vi "RT Positions.vi"(1 "Coordinates":dbl[][](array[numeric]) format="%.6f", 2 "L/R":bool) -> (0 "Cluster":T2)   [LabVIEW 2010]
uses:
  <vilib>/Analysis/Matrix/Datatypes/RealMatrix.ctl
  <vilib>/Analysis/baseanly.llb/Real A x B.vi
  <vilib>/Analysis/NI_AALBase.lvlib
  <vilib>/Analysis/Matrix/NI_Matrix.lvlib
panel:
  out "Humerus rel Trunk":T1
  out "[R]T Trunk":dbl[][](array[numeric])
  out "[R] Trunk":dbl[][](array[numeric])
  out "[R]T Forearm":dbl[][](array[numeric])
  out "[R] Forearm":dbl[][](array[numeric])
  out "[R]T Humerus":dbl[][](array[numeric])
  out "[R] Humerus":dbl[][](array[numeric])
  out "EJC Coord":dbl[](array[numeric])
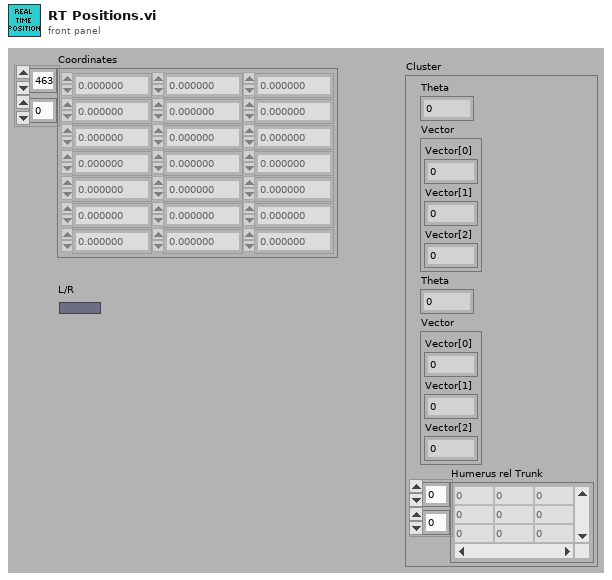
[diagram p1: front panel]
types:
  T1 = typedef "NI_Matrix.lvlib/RealMatrix.ctl" = dbl[][]
  T2 = cluster{"Theta":dbl, "Vector":cluster{"Vector[0]":ext, "Vector[1]":ext, "Vector[2]":ext}, "Theta":dbl, "Vector":cluster{"Vector[0]":ext, "Vector[1]":ext, "Vector[2]":ext}, "Humerus rel Trunk":T1}
  T3 = cluster{"Vector[0]":ext, "Vector[1]":ext, "Vector[2]":ext}
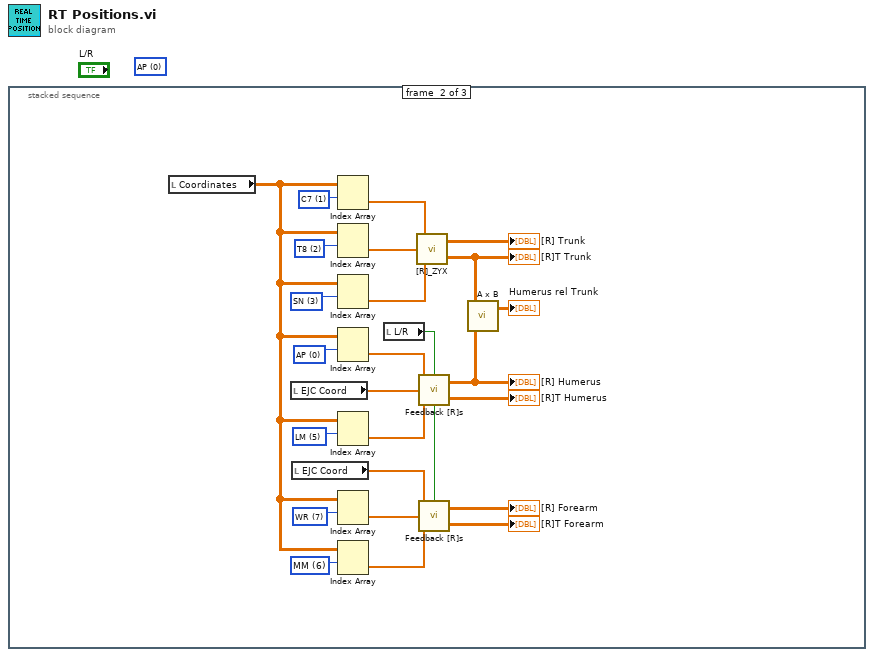
[diagram p0: block diagram]
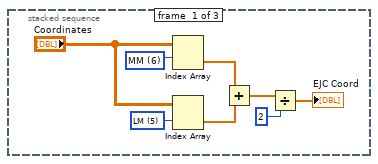
[diagram p2: hidden frame]
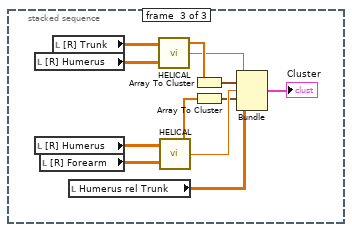
[diagram p3: hidden frame]
diagram:
  (unwired) u16 0 items=["AP", "C7", "T8", "SN", "XP", "LM", "MM", "WR"] ("Marker Names")
  n1 = stacked-sequence {
    frame #0 {
      w7 = u16 5 items=["AP", "C7", "T8", "SN", "XP", "LM", "MM", "WR"] ("Marker Names")
      w8 = u16 6 items=["AP", "C7", "T8", "SN", "XP", "LM", "MM", "WR"] ("Marker Names")
      n2 = Index Array(array="Coordinates", index (row)=w8) -> (element=w6:dbl[])  [unwired: 1 in]
      n3 = Index Array(array="Coordinates", index (row)=w7) -> (element=w5:dbl[])  [unwired: 1 in]
      n4 = Add(x=w6, y=w5) -> (x+y=w4:dbl[])
      n5 = Divide(x=w4, y=2) -> (x/y=→"EJC Coord":dbl[])
    }
    frame #1 {
      w24 = u16 3 items=["AP", "C7", "T8", "SN", "XP", "LM", "MM", "WR"] ("Marker Names")
      w14 = u16 1 items=["AP", "C7", "T8", "SN", "XP", "LM", "MM", "WR"] ("Marker Names")
      w13 = u16 2 items=["AP", "C7", "T8", "SN", "XP", "LM", "MM", "WR"] ("Marker Names")
      w29 = u16 6 items=["AP", "C7", "T8", "SN", "XP", "LM", "MM", "WR"] ("Marker Names")
      w28 = u16 7 items=["AP", "C7", "T8", "SN", "XP", "LM", "MM", "WR"] ("Marker Names")
      w32 = u16 5 items=["AP", "C7", "T8", "SN", "XP", "LM", "MM", "WR"] ("Marker Names")
      w33 = u16 0 items=["AP", "C7", "T8", "SN", "XP", "LM", "MM", "WR"] ("Marker Names")
      n6 = local read "Coordinates"() -> (w20:dbl[][])
      n7 = local read "EJC Coord"() -> (w19:dbl[])
      n8 = local read "EJC Coord"() -> (w16:dbl[])
      n9 = Index Array(array=w20, index (row)=w14) -> (element=w23:dbl[])  [unwired: 1 in]
      n10 = Index Array(array=w20, index (row)=w13) -> (element=w15:dbl[])  [unwired: 1 in]
      n11 = Index Array(array=w20, index (row)=w24) -> (element=w22:dbl[])  [unwired: 1 in]
      n12 = Index Array(array=w20, index (row)=w33) -> (element=w18:dbl[])  [unwired: 1 in]
      n13 = Index Array(array=w20, index (row)=w32) -> (element=w31:dbl[])  [unwired: 1 in]
      n14 = Index Array(array=w20, index (row)=w28) -> (element=w17:dbl[])  [unwired: 1 in]
      n15 = Index Array(array=w20, index (row)=w29) -> (element=w30:dbl[])  [unwired: 1 in]
      n16 = local read "L/R"() -> (w12:bool)
      n17 = call "[R]_ZYX.vi"("Marker 2"=w22, "Origin"=w15, "Marker 1"=w23) -> ("[R]T"=w11:dbl[][], "[R]"=→"[R] Trunk":dbl[][])
      "[R]T Trunk" <- w11
      n18 = call "Feedback [R]s.vi"("L/R"=w12, "Marker 2"=w31, "Origin"=w19, "Marker 1"=w18) -> ("[R]T"=→"[R]T Humerus":dbl[][], "[R]"=w10:dbl[][])
      "[R] Humerus" <- w10
      n19 = call "Feedback [R]s.vi"("L/R"=w12, "Marker 2"=w30, "Origin"=w17, "Marker 1"=w16) -> ("[R]T"=→"[R]T Forearm":dbl[][], "[R]"=→"[R] Forearm":dbl[][])
      n20 = call-poly <vilib>:"A x B.vi"("B"=w10, "A"=w11) -> ("A x B"=→"Humerus rel Trunk":T1)  [unwired: 1 out]
    }
    frame #2 {
      n21 = local read "[R] Humerus"() -> (w40:dbl[][])
      n22 = local read "[R] Humerus"() -> (w37:dbl[][])
      n23 = local read "[R] Forearm"() -> (w45:dbl[][])
      n24 = local read "[R] Trunk"() -> (w38:dbl[][])
      n25 = local read "Humerus rel Trunk"() -> (w39:T1)
      n26 = call "HELICAL.VI"("Proximal\nRotation Matrix"=w38, "Distal Rotation Matrix"=w40) -> ("Vector"=w44:ext[], "Theta"=w43:dbl)  [unwired: 1 out]
      n27 = call "HELICAL.VI"("Proximal\nRotation Matrix"=w37, "Distal Rotation Matrix"=w45) -> ("Vector"=w42:ext[], "Theta"=w41:dbl)  [unwired: 1 out]
      n28 = Array To Cluster(array=w44) -> (cluster=w36:T3)
      n29 = Array To Cluster(array=w42) -> (cluster=w35:T3)
      n30 = Bundle("Theta"=w43, "Vector"=w36, "Theta"=w41, "Vector"=w35, "Humerus rel Trunk"=w39) -> (→"Cluster":T2)  [unwired: 1 in]
    }
  }
